vi "Lab Panel V5.27.vi"() -> ()   [LabVIEW 2013] (continued)
                    n2900 = event-data() -> ()  [unwired: 1 in, 6 out]
                    n2901 = Open/Create/Replace File(file path (use dialog)=w5224, operation (0:open)=T17."replace or create") -> (refnum out=w5230:refnum<file>, error out=w5229:errorcluster)  [unwired: 4 in, 1 out]
                    n2902 = Write to Binary File(file (use dialog)=w5230, data=w5225, error in=w5229) -> (refnum out=w5228:refnum<file>, error out=w5227:errorcluster)  [unwired: 3 in, 1 out]
                    n2903 = Close File(refnum=w5228, error in=w5227) -> (error out=w5226:errorcluster)  [unwired: 1 out]
                    n2904 = local write "data file error"(w5226) -> ()
                  }
                  event "MAIL SETTINGS.OUT SERVER ADDRESS", "MAIL SETTINGS.FROM ACCOUNT", "MAIL SETTINGS.USER NAME", "MAIL SETTINGS.PASSWORD", "Auto Mail Send", "TO (string):": Value Change {
                    n2905 = event-data() -> ()  [unwired: 1 in, 6 out]
                    n2906 = local read "MAIL SETTINGS"() -> (w5235:T7)
                    n2907 = local read "Auto Mail Send"() -> (w5233:bool)
                    n2908 = local read "TO (string):"() -> (w5232:string)
                    n2909 = Open/Create/Replace File(file path (use dialog)=w5236, operation (0:open)=T17."replace or create") -> (refnum out=w5241:refnum<file>, error out=w5240:errorcluster)  [unwired: 4 in, 1 out]
                    n2910 = Bundle("MAIL SETTINGS"=w5235, "Auto Mail Send"=w5233, "TO (string):"=w5232) -> (w5234:T43)  [unwired: 1 in]
                    n2911 = Write to Binary File(file (use dialog)=w5241, data=w5234, error in=w5240) -> (refnum out=w5239:refnum<file>, error out=w5238:errorcluster)  [unwired: 3 in, 1 out]
                    n2912 = Close File(refnum=w5239, error in=w5238) -> (error out=w5237:errorcluster)  [unwired: 1 out]
                    n2913 = local write "data file error"(w5237) -> ()
                  }
                }
              }
            }
          }
          frame #19 {
            # "mail control"
            n2914 = local read "MAIL SETTINGS"() -> (w5258:T7)
            n2915 = local read "Auto Mail Send"() -> (w5244:bool)
            n2916 = Unbundle(w5258) -> ("OUT SERVER ADDRESS"=w5257:string, "FROM ACCOUNT"=w5256:string, "TEST MAIL"=w5255:bool)  [unwired: 4 out]
            n2917 = stacked-sequence {
              tunnel: "TO (string):" -> [_ w5297]
              tunnel: w5258 -> [w5263 w5296]
              tunnel: w5257 -> [w5262 w5295]
              tunnel: w5256 -> [w5261 w5294]
              tunnel: w5255 -> [w5260 _]
              tunnel: w5244 -> [_ w5293]
              tunnel: w5254 -> [_ w5292]
              tunnel: w5253 -> [_ w5291]
              tunnel: w5252 -> [_ w5290]
              tunnel: w5251 -> [_ w5289]
              tunnel: w5250 -> [_ w5288]
              tunnel: w5249 -> [_ w5287]
              tunnel: w5248 -> [_ w5286]
              tunnel: w5247 -> [_ w5285]
              tunnel: w5246 -> [_ w5284]
              tunnel: w5245 -> [_ w5283]
              tunnel: "TO (string):" -> [w5259 _]
              frame #0 {
                # "mail test"
                n2918 = case shown="True" w5260 {
                  tunnel: w5263 -> [_ w5267]
                  tunnel: w5259 -> [_ w5266]
                  tunnel: w5262 -> [_ w5265]
                  tunnel: w5261 -> [_ w5264]
                  frame False {
                  }
                  frame True {
                    n2919 = stacked-sequence {
                      seq-local: [_ _ w5277 _] -> [_ _ _ w5278]
                      tunnel: w5267 -> [w5270 _ _ w5282]
                      tunnel: w5266 -> [_ _ w5275 _]
                      tunnel: w5265 -> [_ _ w5273 _]
                      tunnel: w5264 -> [_ _ w5274 _]
                      frame #0 {
                        n2920 = Bundle(cluster=w5270, "TEST MAIL STATUS"="TEST START") -> (w5268:T7)  [unwired: 6 in]
                        n2921 = local write "MAIL SETTINGS"(w5268) -> ()
                      }
                      frame #1 {
                        n2922 = Wait (ms)(milliseconds to wait=500) -> ()  [unwired: 1 out]
                      }
                      frame #2 {
                        n2923 = call "sub vi - send mail v5.vi"("TO:"=w5275, "subject"="MAIL TEST FROM LAB PANEL", "from"=w5274, "out going server"=w5273, "message"="TEST MESSAGE") -> ("error out"=w5277:errorcluster)  [unwired: 10 in]
                      }
                      frame #3 {
                        n2924 = Bundle(cluster=w5282, "TEST MAIL"=FALSE, "TEST MAIL STATUS"="TEST END", "mail error"=w5278) -> (w5280:T7)  [unwired: 4 in]
                        n2925 = local write "MAIL SETTINGS"(w5280) -> ()
                      }
                    }
                  }
                }
              }
              frame #1 {
                # "mail report"
                n2926 = stacked-sequence {
                  seq-local: [_ w5340 _ _] -> [_ _ _ w5530]
                  seq-local: [_ _ w5443 _] -> [_ _ _ w5520]
                  seq-local: [w5307 _ _ _] -> [_ w5357 _ _]
                  seq-local: [w5306 _ _ _] -> [_ w5356 _ _]
                  seq-local: [w5304 _ _ _] -> [_ w5354 _ _]
                  seq-local: [w5305 _ _ _] -> [_ w5355 _ _]
                  seq-local: [w5303 _ _ _] -> [_ w5353 _ _]
                  seq-local: [w5302 _ _ _] -> [_ w5348 _ _]
                  seq-local: [w5301 _ _ _] -> [_ w5349 _ _]
                  seq-local: [w5300 _ _ _] -> [_ w5350 _ _]
                  seq-local: [w5299 _ _ _] -> [_ w5351 _ _]
                  seq-local: [w5298 _ _ _] -> [_ w5352 _ _]
                  tunnel: w5297 -> [_ _ _ w5531]
                  tunnel: w5296 -> [_ _ _ w5514]
                  tunnel: w5295 -> [_ _ _ w5528]
                  tunnel: w5294 -> [_ _ _ w5527]
                  tunnel: w5293 -> [w5338 _ _ w5522]
                  tunnel: w5292 -> [_ _ w5473 _]
                  tunnel: w5291 -> [_ _ w5470 _]
                  tunnel: w5290 -> [_ _ w5469 _]
                  tunnel: w5289 -> [_ _ w5468 _]
                  tunnel: w5288 -> [_ _ w5467 _]
                  tunnel: w5287 -> [_ _ w5466 _]
                  tunnel: w5286 -> [_ _ w5465 _]
                  tunnel: w5285 -> [_ _ w5464 _]
                  tunnel: w5284 -> [_ _ w5463 _]
                  tunnel: w5283 -> [_ _ w5462 _]
                  frame #0 {
                    n2927 = case shown="False" w5338 {
                      frame False {
                        n2928 = local write "mail control"("") -> ()
                      }
                      frame True {
                      }
                    }
                    n2929 = local read "SET LAB01-1"() -> (w5337:T5)
                    n2930 = local read "SET LAB01-2"() -> (w5336:T5)
                    n2931 = local read "SET LAB02-1"() -> (w5335:T5)
                    n2932 = local read "SET LAB02-2"() -> (w5334:T5)
                    n2933 = local read "SET LAB03-1"() -> (w5333:T5)
                    n2934 = local read "SET LAB04-1"() -> (w5331:T5)
                    n2935 = local read "SET LAB05-1"() -> (w5329:T5)
                    n2936 = local read "SET LAB03-2"() -> (w5332:T5)
                    n2937 = local read "SET LAB04-2"() -> (w5330:T5)
                    n2938 = local read "SET LAB05-2"() -> (w5328:T5)
                    n2939 = Unbundle(w5333) -> ("DESCRIPTION"=w5313:string)  [unwired: 4 out]
                    n2940 = Unbundle(w5332) -> ("DESCRIPTION"=w5312:string)  [unwired: 4 out]
                    n2941 = Unbundle(w5331) -> ("DESCRIPTION"=w5311:string)  [unwired: 4 out]
                    n2942 = Unbundle(w5328) -> ("DESCRIPTION"=w5308:string)  [unwired: 4 out]
                    n2943 = Unbundle(w5334) -> ("DESCRIPTION"=w5314:string)  [unwired: 4 out]
                    n2944 = Unbundle(w5330) -> ("DESCRIPTION"=w5310:string)  [unwired: 4 out]
                    n2945 = Unbundle(w5337) -> ("DESCRIPTION"=w5326:string)  [unwired: 4 out]
                    n2946 = Unbundle(w5335) -> ("DESCRIPTION"=w5315:string)  [unwired: 4 out]
                    n2947 = Unbundle(w5329) -> ("DESCRIPTION"=w5309:string)  [unwired: 4 out]
                    n2948 = Unbundle(w5336) -> ("DESCRIPTION"=w5316:string)  [unwired: 4 out]
                    n2949 = Concatenate Strings("[LAB05-2/", w5308) -> (w5298:string)
                    n2950 = Concatenate Strings("[LAB05-1/", w5309) -> (w5299:string)
                    n2951 = Concatenate Strings("[LAB04-2/", w5310) -> (w5300:string)
                    n2952 = Concatenate Strings("[LAB03-2/", w5312) -> (w5302:string)
                    n2953 = Concatenate Strings("[LAB04-1/", w5311) -> (w5301:string)
                    n2954 = Concatenate Strings("[LAB03-1/", w5313) -> (w5303:string)
                    n2955 = Concatenate Strings("[LAB01-2/", w5316) -> (w5306:string)
                    n2956 = Concatenate Strings("[LAB02-2/", w5314) -> (w5304:string)
                    n2957 = Concatenate Strings("[LAB01-1/", w5326) -> (w5307:string)
                    n2958 = Concatenate Strings("[LAB02-1/", w5315) -> (w5305:string)
                  }
                  frame #1 {
                    w5361 = "/"
                    w5362 = 2.0
                    n2959 = local read "DISP LAB01-2"() -> (w5441:T4)
                    n2960 = local read "DISP LAB01-1"() -> (w5442:T4)
                    n2961 = local read "DISP LAB02-1"() -> (w5440:T4)
                    n2962 = local read "DISP LAB03-2"() -> (w5437:T4)
                    n2963 = local read "DISP LAB02-2"() -> (w5439:T4)
                    n2964 = local read "DISP LAB03-1"() -> (w5438:T4)
                    n2965 = local read "DISP LAB04-2"() -> (w5435:T4)
                    n2966 = local read "DISP LAB04-1"() -> (w5436:T4)
                    n2967 = local read "DISP LAB05-1"() -> (w5434:T4)
                    n2968 = local read "DISP LAB05-2"() -> (w5433:T4)
                    n2969 = Unbundle(w5441) -> ("CYCLE"=w5425:dbl, "MINS"=w5424:dbl, "STATUS"=w5421:string)
                    n2970 = Unbundle(w5442) -> ("CYCLE"=w5430:dbl, "MINS"=w5429:dbl, "STATUS"=w5426:string)
                    n2971 = Unbundle(w5440) -> ("CYCLE"=w5418:dbl, "MINS"=w5417:dbl, "STATUS"=w5416:string)
                    n2972 = Unbundle(w5437) -> ("CYCLE"=w5405:dbl, "MINS"=w5404:dbl, "STATUS"=w5401:string)
                    n2973 = Unbundle(w5438) -> ("CYCLE"=w5410:dbl, "MINS"=w5409:dbl, "STATUS"=w5406:string)
                    n2974 = Unbundle(w5439) -> ("CYCLE"=w5415:dbl, "MINS"=w5414:dbl, "STATUS"=w5411:string)
                    n2975 = Unbundle(w5436) -> ("CYCLE"=w5400:dbl, "MINS"=w5399:dbl, "STATUS"=w5396:string)
                    n2976 = Unbundle(w5435) -> ("CYCLE"=w5395:dbl, "MINS"=w5394:dbl, "STATUS"=w5391:string)
                    n2977 = Unbundle(w5434) -> ("CYCLE"=w5390:dbl, "MINS"=w5389:dbl, "STATUS"=w5386:string)
                    n2978 = Unbundle(w5433) -> ("CYCLE"=w5432:dbl, "MINS"=w5431:dbl, "STATUS"=w5383:string)
                    n2979 = Number To Decimal String(number=w5418) -> (decimal integer string=w5420:string)  [unwired: 1 in]
                    n2980 = Number To Decimal String(number=w5415) -> (decimal integer string=w5413:string)  [unwired: 1 in]
                    n2981 = Number To Decimal String(number=w5410) -> (decimal integer string=w5408:string)  [unwired: 1 in]
                    n2982 = Number To Decimal String(number=w5425) -> (decimal integer string=w5423:string)  [unwired: 1 in]
                    n2983 = Number To Decimal String(number=w5405) -> (decimal integer string=w5403:string)  [unwired: 1 in]
                    n2984 = Number To Decimal String(number=w5430) -> (decimal integer string=w5428:string)  [unwired: 1 in]
                    n2985 = Number To Decimal String(number=w5432) -> (decimal integer string=w5385:string)  [unwired: 1 in]
                    n2986 = Number To Decimal String(number=w5400) -> (decimal integer string=w5398:string)  [unwired: 1 in]
                    n2987 = Number To Decimal String(number=w5395) -> (decimal integer string=w5393:string)  [unwired: 1 in]
                    n2988 = Number To Decimal String(number=w5390) -> (decimal integer string=w5388:string)  [unwired: 1 in]
                    n2989 = Number To Fractional String(number=w5417, precision (6)=w5362) -> (F-format string=w5419:string)  [unwired: 2 in]
                    n2990 = Number To Fractional String(number=w5404, precision (6)=w5362) -> (F-format string=w5402:string)  [unwired: 2 in]
                    n2991 = Number To Fractional String(number=w5414, precision (6)=w5362) -> (F-format string=w5412:string)  [unwired: 2 in]
                    n2992 = Number To Fractional String(number=w5409, precision (6)=w5362) -> (F-format string=w5407:string)  [unwired: 2 in]
                    n2993 = Number To Fractional String(number=w5394, precision (6)=w5362) -> (F-format string=w5392:string)  [unwired: 2 in]
                    n2994 = Number To Fractional String(number=w5399, precision (6)=w5362) -> (F-format string=w5397:string)  [unwired: 2 in]
                    n2995 = Number To Fractional String(number=w5424, precision (6)=w5362) -> (F-format string=w5422:string)  [unwired: 2 in]
                    n2996 = Number To Fractional String(number=w5389, precision (6)=w5362) -> (F-format string=w5387:string)  [unwired: 2 in]
                    n2997 = Number To Fractional String(number=w5429, precision (6)=w5362) -> (F-format string=w5427:string)  [unwired: 2 in]
                    n2998 = Number To Fractional String(number=w5431, precision (6)=w5362) -> (F-format string=w5384:string)  [unwired: 2 in]
                    n2999 = Concatenate Strings(w5361, w5403, w5361, w5402, w5361, w5401) -> (w5377:string)
                    n3000 = Concatenate Strings(w5361, w5398, w5361, w5397, w5361, w5396) -> (w5376:string)
                    n3001 = Concatenate Strings(w5361, w5393, w5361, w5392, w5361, w5391) -> (w5375:string)
                    n3002 = Concatenate Strings(w5361, w5388, w5361, w5387, w5361, w5386) -> (w5374:string)
                    n3003 = Concatenate Strings(w5361, w5385, w5361, w5384, w5361, w5383) -> (w5373:string)
                    n3004 = Concatenate Strings(w5361, w5428, w5361, w5427, w5361, w5426) -> (w5382:string)
                    n3005 = Concatenate Strings(w5361, w5408, w5361, w5407, w5361, w5406) -> (w5378:string)
                    n3006 = Concatenate Strings(w5361, w5423, w5361, w5422, w5361, w5421) -> (w5381:string)
                    n3007 = Concatenate Strings(w5361, w5420, w5361, w5419, w5361, w5416) -> (w5380:string)
                    n3008 = Concatenate Strings(w5361, w5413, w5361, w5412, w5361, w5411) -> (w5379:string)
                    n3009 = Concatenate Strings("]", "\r") -> (w5358:string)
                    n3010 = Concatenate Strings(w5353, w5378, w5358) -> (w5368:string)
                    n3011 = Concatenate Strings(w5355, w5380, w5358) -> (w5370:string)
                    n3012 = Concatenate Strings(w5354, w5379, w5358) -> (w5369:string)
                    n3013 = Concatenate Strings(w5350, w5375, w5358) -> (w5365:string)
                    n3014 = Concatenate Strings(w5351, w5374, w5358) -> (w5366:string)
                    n3015 = Concatenate Strings(w5349, w5376, w5358) -> (w5364:string)
                    n3016 = Concatenate Strings(w5348, w5377, w5358) -> (w5363:string)
                    n3017 = Concatenate Strings(w5352, w5373, w5358) -> (w5367:string)
                    n3018 = Concatenate Strings(w5356, w5381, w5358) -> (w5371:string)
                    n3019 = Concatenate Strings(w5357, w5382, w5358) -> (w5372:string)
                    n3020 = Concatenate Strings(w5372, w5371, w5370, w5369, w5368, w5363, w5364, w5365, w5366, w5367) -> (w5341:string)
                    n3021 = Concatenate Strings("[PANEL/", "DESC/", "CYCLES/", "MINS/", "STATUS]", "\r", w5341) -> (w5340:string)
                    "MAIL REPORT" <- w5340
                    n3022 = global write "Global display 3.vi" "log all"(w5340) -> ()
                  }
                  frame #2 {
                    w5471 = "END"
                    n3023 = local read "mail control"() -> (w5472:string)
                    n3024 = case shown="False" w5467 {
                      tunnel: w5472 -> [w5496 _]
                      tunnel: w5471 -> [w5495 _]
                      tunnel: [w5494 FALSE] -> w5457
                      frame False {
                        n3025 = Equal?(x=w5496, y=w5495) -> (x = y?=w5494:bool)
                      }
                      frame True {
                      }
                    }
                    n3026 = case shown="False" w5473 {
                      tunnel: w5472 -> [w5512 _]
                      tunnel: w5471 -> [w5511 _]
                      tunnel: [w5510 FALSE] -> w5461
                      frame False {
                        n3027 = Equal?(x=w5512, y=w5511) -> (x = y?=w5510:bool)
                      }
                      frame True {
                      }
                    }
                    n3028 = case shown="False" w5470 {
                      tunnel: w5472 -> [w5508 _]
                      tunnel: w5471 -> [w5507 _]
                      tunnel: [w5506 FALSE] -> w5460
                      frame False {
                        n3029 = Equal?(x=w5508, y=w5507) -> (x = y?=w5506:bool)
                      }
                      frame True {
                      }
                    }
                    n3030 = case shown="False" w5468 {
                      tunnel: w5472 -> [w5500 _]
                      tunnel: w5471 -> [w5499 _]
                      tunnel: [w5498 FALSE] -> w5458
                      frame False {
                        n3031 = Equal?(x=w5500, y=w5499) -> (x = y?=w5498:bool)
                      }
                      frame True {
                      }
                    }
                    n3032 = case shown="False" w5469 {
                      tunnel: w5472 -> [w5504 _]
                      tunnel: w5471 -> [w5503 _]
                      tunnel: [w5502 FALSE] -> w5459
                      frame False {
                        n3033 = Equal?(x=w5504, y=w5503) -> (x = y?=w5502:bool)
                      }
                      frame True {
                      }
                    }
                    n3034 = Or(x=w5459, y=w5458) -> (x .or. y?=w5450:bool)
                    n3035 = Or(x=w5461, y=w5460) -> (x .or. y?=w5451:bool)
                    n3036 = Or(x=w5451, y=w5450) -> (x .or. y?=w5446:bool)
                    n3037 = case shown="False" w5463 {
                      tunnel: w5472 -> [w5480 _]
                      tunnel: w5471 -> [w5479 _]
                      tunnel: [w5478 FALSE] -> w5452
                      frame False {
                        n3038 = Equal?(x=w5480, y=w5479) -> (x = y?=w5478:bool)
                      }
                      frame True {
                      }
                    }
                    n3039 = case shown="False" w5462 {
                      tunnel: w5472 -> [w5476 _]
                      tunnel: w5471 -> [w5475 _]
                      tunnel: [w5474 FALSE] -> w5456
                      frame False {
                        n3040 = Equal?(x=w5476, y=w5475) -> (x = y?=w5474:bool)
                      }
                      frame True {
                      }
                    }
                    n3041 = case shown="False" w5464 {
                      tunnel: w5472 -> [w5484 _]
                      tunnel: w5471 -> [w5483 _]
                      tunnel: [w5482 FALSE] -> w5453
                      frame False {
                        n3042 = Equal?(x=w5484, y=w5483) -> (x = y?=w5482:bool)
                      }
                      frame True {
                      }
                    }
                    n3043 = case shown="False" w5466 {
                      tunnel: w5472 -> [w5492 _]
                      tunnel: w5471 -> [w5491 _]
                      tunnel: [w5490 FALSE] -> w5455
                      frame False {
                        n3044 = Equal?(x=w5492, y=w5491) -> (x = y?=w5490:bool)
                      }
                      frame True {
                      }
                    }
                    n3045 = case shown="False" w5465 {
                      tunnel: w5472 -> [w5488 _]
                      tunnel: w5471 -> [w5487 _]
                      tunnel: [w5486 FALSE] -> w5454
                      frame False {
                        n3046 = Equal?(x=w5488, y=w5487) -> (x = y?=w5486:bool)
                      }
                      frame True {
                      }
                    }
                    n3047 = Or(x=w5455, y=w5454) -> (x .or. y?=w5449:bool)
                    n3048 = Or(x=w5453, y=w5452) -> (x .or. y?=w5448:bool)
                    n3049 = Or(x=w5456, y=w5457) -> (x .or. y?=w5444:bool)
                    n3050 = Or(x=w5449, y=w5448) -> (x .or. y?=w5447:bool)
                    n3051 = Or(x=w5446, y=w5447) -> (x .or. y?=w5445:bool)
                    n3052 = Or(x=w5445, y=w5444) -> (x .or. y?=w5443:bool)
                  }
                  frame #3 {
                    n3053 = local read "on loops"() -> (w5526:dbl)
                    n3054 = local read "jig cycle"() -> (w5523:dbl)
                    n3055 = local read "Send Mail Now"() -> (w5517:bool)
                    n3056 = Add(x=w5526, y=5.0) -> (x+y=w5524:dbl)
                    n3057 = Equal?(x=w5523, y=w5524) -> (x = y?=w5518:bool)
                    n3058 = And(x=w5518, y=w5517) -> (x .and. y?=w5516:bool)
                    n3059 = And(x=w5522, y=w5518) -> (x .and. y?=w5521:bool)
                    n3060 = And(x=w5521, y=w5520) -> (x .and. y?=w5519:bool)
                    n3061 = Or(x=w5519, y=w5516) -> (x .or. y?=w5515:bool)
                    n3062 = case shown="True" w5515 {
                      tunnel: w5531 -> [_ w5537]
                      tunnel: w5530 -> [_ w5536]
                      tunnel: "Lab Panel Test Status" -> [_ w5535]
                      tunnel: w5528 -> [_ w5534]
                      tunnel: w5527 -> [_ w5533]
                      tunnel: w5514 -> [_ w5532]
                      frame False {
                      }
                      frame True {
                        n3063 = stacked-sequence {
                          tunnel: w5537 -> [w5546 _]
                          tunnel: w5536 -> [w5545 _]
                          tunnel: w5535 -> [w5544 _]
                          tunnel: w5534 -> [w5543 _]
                          tunnel: w5533 -> [w5542 _]
                          tunnel: w5532 -> [w5541 _]
                          frame #0 {
                            n3064 = call "sub vi - send mail v5.vi"("TO:"=w5546, "subject"=w5544, "Info"="Test station status report", "from"=w5542, "out going server"=w5543, "message"=w5545) -> ("error out"=w5540:errorcluster)  [unwired: 9 in]
                            n3065 = Bundle(cluster=w5541, "mail error"=w5540) -> (w5539:T7)  [unwired: 6 in]
                            n3066 = local write "MAIL SETTINGS"(w5539) -> ()
                          }
                          frame #1 {
                            n3067 = local write "mail control"("") -> ()
                            n3068 = local write "Send Mail Now"(FALSE) -> ()
                          }
                        }
                      }
                    }
                  }
                }
              }
            }
          }
          frame #20 {
            # "save jig cycle values once all run switches are off"
            n3069 = stacked-sequence {
              tunnel: w5558 -> [_ w5587]
              tunnel: w5557 -> [_ w5586]
              tunnel: w5556 -> [_ w5585]
              tunnel: w5555 -> [_ w5584]
              tunnel: w5554 -> [_ w5583]
              tunnel: w5553 -> [_ w5582]
              tunnel: w5552 -> [_ w5581]
              tunnel: w5551 -> [_ w5580]
              tunnel: w5550 -> [_ w5579]
              tunnel: w5549 -> [_ w5578]
              frame #0 {
              }
              frame #1 {
                n3070 = Not(x=w5578) -> (.not. x?=w5561:bool)
                n3071 = Not(x=w5586) -> (.not. x?=w5576:bool)
                n3072 = Not(x=w5583) -> (.not. x?=w5571:bool)
                n3073 = Not(x=w5581) -> (.not. x?=w5567:bool)
                n3074 = Not(x=w5579) -> (.not. x?=w5563:bool)
                n3075 = Not(x=w5587) -> (.not. x?=w5577:bool)
                n3076 = Not(x=w5585) -> (.not. x?=w5575:bool)
                n3077 = Not(x=w5582) -> (.not. x?=w5569:bool)
                n3078 = Not(x=w5584) -> (.not. x?=w5573:bool)
                n3079 = Not(x=w5580) -> (.not. x?=w5565:bool)
                n3080 = local read "Save JC"() -> (w5589:bool)
                n3081 = And(x=w5577, y=w5576) -> (x .and. y?=w5574:bool)
                n3082 = And(x=w5574, y=w5575) -> (x .and. y?=w5572:bool)
                n3083 = And(x=w5572, y=w5573) -> (x .and. y?=w5570:bool)
                n3084 = And(x=w5570, y=w5571) -> (x .and. y?=w5568:bool)
                n3085 = And(x=w5568, y=w5569) -> (x .and. y?=w5566:bool)
                n3086 = And(x=w5566, y=w5567) -> (x .and. y?=w5564:bool)
                n3087 = And(x=w5564, y=w5565) -> (x .and. y?=w5562:bool)
                n3088 = And(x=w5562, y=w5563) -> (x .and. y?=w5560:bool)
                n3089 = And(x=w5560, y=w5561) -> (x .and. y?=w5559:bool)
                n3090 = And(x=w5559, y=w5589) -> (x .and. y?=w5588:bool)
                n3091 = case shown="True" w5588 {
                  tunnel: w5559 -> [w5590 _]
                  frame False {
                    n3092 = case shown="False" w5590 {
                      frame False {
                        n3093 = local write "Save JC"(TRUE) -> ()
                      }
                      frame True {
                      }
                    }
                  }
                  frame True {
                    n3094 = stacked-sequence {
                      frame #0 {
                        n3095 = String To Path(string="c:\\crabtree\\Jig Cycles\\") -> (path=w5602:path)
                        n3096 = Build Path(base path=w5602, name or relative path="jigcycles.bin") -> (appended path=w5600:path)
                        n3097 = Create Folder(path (use dialog)=w5602) -> (error out=w5604:errorcluster)  [unwired: 2 in, 2 out]
                        n3098 = local read "JIG RELAY CYCLES"() -> (w5594:T8)
                        n3099 = call <vilib>:"Clear Errors.vi"("error in (no error)"=w5604) -> ()  [unwired: 6 in, 1 out]
                        n3100 = local write "Save JC"(FALSE) -> ()
                        n3101 = Open/Create/Replace File(file path (use dialog)=w5600, operation (0:open)=T17."replace or create") -> (refnum out=w5598:refnum<file>, error out=w5599:errorcluster)  [unwired: 4 in, 1 out]
                        n3102 = Write to Binary File(file (use dialog)=w5598, data=w5594, error in=w5599) -> (refnum out=w5597:refnum<file>, error out=w5596:errorcluster)  [unwired: 3 in, 1 out]
                        n3103 = Close File(refnum=w5597, error in=w5596) -> (error out=w5595:errorcluster)  [unwired: 1 out]
                        n3104 = local write "data file error"(w5595) -> ()
                      }
                      frame #1 {
                        n3105 = local read "JIG RELAY CYCLES"() -> (w5627:T8)
                        n3106 = Unbundle By Name(w5627) -> ("LAB01-1"=w5622:dbl, "LAB01-2"=w5621:dbl, "LAB02-1"=w5619:dbl, "LAB02-2"=w5618:dbl, "LAB03-1"=w5616:dbl, "LAB03-2"=w5613:dbl, "LAB04-1"=w5612:dbl, "LAB04-2"=w5610:dbl, "LAB05-1"=w5608:dbl, "LAB05-2"=w5606:dbl)
                        n3107 = stacked-sequence {
                          tunnel: w5622 -> [w5630 _ _ _ _ _ _ _ _ _]
                          tunnel: 1000000 -> [w5633 w5643 w5653 w5663 w5673 w5683 w5693 w5703 w5713 w5723]
                          tunnel: [w5631 _ _ _ _ _ _ _ _ _] -> w5625
                          tunnel: "TEST STATION HAS REACHED 1 MILLION CYCLES, REPLACE  CONTROL RELAYS" -> [w5629 w5641 w5651 w5661 w5671 w5681 w5691 w5701 w5711 w5721]
                          tunnel: [_ w5640 _ _ _ _ _ _ _ _] -> w5623
                          tunnel: w5621 -> [_ w5639 _ _ _ _ _ _ _ _]
                          tunnel: [_ _ w5650 _ _ _ _ _ _ _] -> w5620
                          tunnel: w5619 -> [_ _ w5649 _ _ _ _ _ _ _]
                          tunnel: w5618 -> [_ _ _ w5660 _ _ _ _ _ _]
                          tunnel: [_ _ _ w5659 _ _ _ _ _ _] -> w5617
                          tunnel: w5616 -> [_ _ _ _ w5670 _ _ _ _ _]
                          tunnel: [_ _ _ _ w5669 _ _ _ _ _] -> w5615
                          tunnel: [_ _ _ _ _ w5680 _ _ _ _] -> w5614
                          tunnel: w5613 -> [_ _ _ _ _ w5679 _ _ _ _]
                          tunnel: w5612 -> [_ _ _ _ _ _ w5690 _ _ _]
                          tunnel: [_ _ _ _ _ _ w5689 _ _ _] -> w5611
                          tunnel: w5610 -> [_ _ _ _ _ _ _ w5700 _ _]
                          tunnel: [_ _ _ _ _ _ _ w5699 _ _] -> w5609
                          tunnel: w5608 -> [_ _ _ _ _ _ _ _ w5710 _]
                          tunnel: [_ _ _ _ _ _ _ _ w5709 _] -> w5607
                          tunnel: w5606 -> [_ _ _ _ _ _ _ _ _ w5720]
                          tunnel: [_ _ _ _ _ _ _ _ _ w5719] -> w5605
                          frame #0 {
                            n3108 = Greater?(x=w5630, y=w5633) -> (0:w5632:bool)
                            n3109 = case shown="True" w5632 {
                              tunnel: [w5634 0] -> w5631
                              tunnel: w5630 -> [w5634 _]
                              tunnel: w5629 -> [_ w5635]
                              frame False {
                              }
                              frame True {
                                n3110 = Concatenate Strings("LA01-1 ", w5635) -> (w5638:string)
                                n3111 = One Button Dialog(message=w5638) -> ()  [unwired: 1 in, 1 out]
                              }
                            }
                          }
                          frame #1 {
                            n3112 = Greater?(x=w5639, y=w5643) -> (0:w5642:bool)
                            n3113 = case shown="True" w5642 {
                              tunnel: [w5644 0] -> w5640
                              tunnel: w5639 -> [w5644 _]
                              tunnel: w5641 -> [_ w5645]
                              frame False {
                              }
                              frame True {
                                n3114 = Concatenate Strings("LA01-2 ", w5645) -> (w5648:string)
                                n3115 = One Button Dialog(message=w5648) -> ()  [unwired: 1 in, 1 out]
                              }
                            }
                          }
                          frame #2 {
                            n3116 = Greater?(x=w5649, y=w5653) -> (0:w5652:bool)
                            n3117 = case shown="True" w5652 {
                              tunnel: [w5654 0] -> w5650
                              tunnel: w5649 -> [w5654 _]
                              tunnel: w5651 -> [_ w5655]
                              frame False {
                              }
                              frame True {
                                n3118 = Concatenate Strings("LA02-1 ", w5655) -> (w5658:string)
                                n3119 = One Button Dialog(message=w5658) -> ()  [unwired: 1 in, 1 out]
                              }
                            }
                          }
                          frame #3 {
                            n3120 = Greater?(x=w5660, y=w5663) -> (0:w5662:bool)
                            n3121 = case shown="True" w5662 {
                              tunnel: [w5664 0] -> w5659
                              tunnel: w5660 -> [w5664 _]
                              tunnel: w5661 -> [_ w5665]
                              frame False {
                              }
                              frame True {
                                n3122 = Concatenate Strings("LA02-2 ", w5665) -> (w5668:string)
                                n3123 = One Button Dialog(message=w5668) -> ()  [unwired: 1 in, 1 out]
                              }
                            }
                          }
                          frame #4 {
                            n3124 = Greater?(x=w5670, y=w5673) -> (0:w5672:bool)
                            n3125 = case shown="True" w5672 {
                              tunnel: [w5674 0] -> w5669
                              tunnel: w5670 -> [w5674 _]
                              tunnel: w5671 -> [_ w5675]
                              frame False {
                              }
                              frame True {
                                n3126 = Concatenate Strings("LA03-1 ", w5675) -> (w5678:string)
                                n3127 = One Button Dialog(message=w5678) -> ()  [unwired: 1 in, 1 out]
                              }
                            }
                          }
                          frame #5 {
                            n3128 = Greater?(x=w5679, y=w5683) -> (0:w5682:bool)
                            n3129 = case shown="True" w5682 {
                              tunnel: [w5684 0] -> w5680
                              tunnel: w5679 -> [w5684 _]
                              tunnel: w5681 -> [_ w5685]
                              frame False {
                              }
                              frame True {
                                n3130 = Concatenate Strings("LA03-2 ", w5685) -> (w5688:string)
                                n3131 = One Button Dialog(message=w5688) -> ()  [unwired: 1 in, 1 out]
                              }
                            }
                          }
                          frame #6 {
                            n3132 = Greater?(x=w5690, y=w5693) -> (0:w5692:bool)
                            n3133 = case shown="True" w5692 {
                              tunnel: [w5694 0] -> w5689
                              tunnel: w5690 -> [w5694 _]
                              tunnel: w5691 -> [_ w5695]
                              frame False {
                              }
                              frame True {
                                n3134 = Concatenate Strings("LA04-1 ", w5695) -> (w5698:string)
                                n3135 = One Button Dialog(message=w5698) -> ()  [unwired: 1 in, 1 out]
                              }
                            }
                          }
                          frame #7 {
                            n3136 = Greater?(x=w5700, y=w5703) -> (0:w5702:bool)
                            n3137 = case shown="True" w5702 {
                              tunnel: [w5704 0] -> w5699
                              tunnel: w5700 -> [w5704 _]
                              tunnel: w5701 -> [_ w5705]
                              frame False {
                              }
                              frame True {
                                n3138 = Concatenate Strings("LA04-2 ", w5705) -> (w5708:string)
                                n3139 = One Button Dialog(message=w5708) -> ()  [unwired: 1 in, 1 out]
                              }
                            }
                          }
                          frame #8 {
                            n3140 = Greater?(x=w5710, y=w5713) -> (0:w5712:bool)
                            n3141 = case shown="True" w5712 {
                              tunnel: [w5714 0] -> w5709
                              tunnel: w5710 -> [w5714 _]
                              tunnel: w5711 -> [_ w5715]
                              frame False {
                              }
                              frame True {
                                n3142 = Concatenate Strings("LA05-1 ", w5715) -> (w5718:string)
                                n3143 = One Button Dialog(message=w5718) -> ()  [unwired: 1 in, 1 out]
                              }
                            }
                          }
                          frame #9 {
                            n3144 = Greater?(x=w5720, y=w5723) -> (0:w5722:bool)
                            n3145 = case shown="True" w5722 {
                              tunnel: [w5724 0] -> w5719
                              tunnel: w5720 -> [w5724 _]
                              tunnel: w5721 -> [_ w5725]
                              frame False {
                              }
                              frame True {
                                n3146 = Concatenate Strings("LA05-2 ", w5725) -> (w5728:string)
                                n3147 = One Button Dialog(message=w5728) -> ()  [unwired: 1 in, 1 out]
                              }
                            }
                          }
                        }
                        n3148 = Bundle By Name(cluster=w5627, "LAB01-1"=w5625, "LAB01-2"=w5623, "LAB02-1"=w5620, "LAB02-2"=w5617, "LAB03-1"=w5615, "LAB03-2"=w5614, "LAB04-1"=w5611, "LAB04-2"=w5609, "LAB05-1"=w5607, "LAB05-2"=w5605) -> (w5626:T8)
                        n3149 = local write "JIG RELAY CYCLES"(w5626) -> ()
                      }
                    }
                  }
                }
              }
            }
          }
          frame #21 {
            # "get temperature values"
            n3150 = local read "Simulate"() -> (w5741:bool)
            n3151 = local read "Temp Test Cal"() -> (w5738:dbl)
            n3152 = stacked-sequence {
              seq-local: [w5743 _] -> [_ w5788]
              tunnel: w5741 -> [_ w5801]
              tunnel: T14 {"1  (A) cal"=1.0, "1 (V) cal"=1.0, "1 (PF) cal"=1.0, "1 (TL) cal"=1.0, "1 (TN) cal"=1.0, "2 (A) cal"=1.0, "2 (V) cal"=1.0, "2 (PF) cal"=1.0, "2 (TL) cal"=1.0, "2 (TN) cal"=1.0} ("CAL LAB01") -> [_ w5800]
              tunnel: w5739 -> [_ w5799]
              tunnel: w5738 -> [_ w5798]
              tunnel: w5737 -> [_ w5797]
              tunnel: w5736 -> [_ w5796]
              tunnel: w5735 -> [_ w5795]
              tunnel: w5734 -> [_ w5794]
              tunnel: w5733 -> [_ w5793]
              tunnel: w5732 -> [_ w5792]
              tunnel: w5731 -> [_ w5791]
              tunnel: w5730 -> [_ w5790]
              tunnel: w5729 -> [_ w5789]
              frame #0 {
                # "only get temperature from initial valid temperature circuits"
                n3153 = local read "Select COM port"() -> (w5751:refnum<visa-resource-name>)
                "COM port" <- w5751
                n3154 = global write "Global 1.vi" "COM port"(w5751) -> ()
                n3155 = local read "Temp read loop"() -> (w5748:dbl)
                n3156 = global write "Global 1.vi" "tmp dly lps"("Temp Delay Lps") -> ()
                n3157 = global write "Global 1.vi" "dly value"("Temp Value") -> ()
                n3158 = local read "jig cycle"() -> (w5752:dbl)
                n3159 = local read "on loops"() -> (w5754:dbl)
                n3160 = Equal?(x=w5748, y=1) -> (x = y?=w5745:bool)
                n3161 = Add(x=w5754, y=6) -> (x+y=w5755:dbl)
                n3162 = Equal?(x=w5752, y=w5755) -> (x = y?=w5746:bool)
                n3163 = And(x=w5746, y=w5745) -> (x .and. y?=w5744:bool)
                n3164 = Or(x=w5744, y="Read Temp") -> (x .or. y?=w5743:bool)
                n3165 = case shown="True" w5743 {
                  frame False {
                  }
                  frame True {
                    n3166 = local read "Simulate"() -> (w5757:bool)
                    n3167 = local write "TEMP"(TRUE) -> ()
                    n3168 = local write "Read Temp"(FALSE) -> ()
                    n3169 = stacked-sequence {
                      tunnel: 1.0 -> [_ _ _ _ w5787]
                      tunnel: w5757 -> [_ _ _ _ w5786]
                      frame #0 {
                        # "only switch relay on to reset temp circuits if busy testing"
                        n3170 = disable-structure shown="Disabled" {
                          frame Disabled {
                            n3171 = local read "Any Test Running"() -> ()  [unwired: 1 out]
                          }
                          frame Enabled {
                          }
                        }
                        n3172 = local read "USB OUT 0"() -> (w5761:bool[])
                        n3173 = local read "USB OUT 2"() -> (w5763:bool[])
                        n3174 = local read "USB OUT 1"() -> (w5762:bool[])
                        n3175 = Insert Into Array(array=w5763, index=7, new element=TRUE) -> (w5764:bool[])
                        n3176 = call "sub vi - Drive Relays All v6.vi"("Array #2"=w5764, "Array #1"=w5762, "Array #0"=w5761) -> ()  [unwired: 8 in, 1 out]
                      }
                      frame #1 {
                        # "time delay"
                        n3177 = Wait (ms)(milliseconds to wait=500) -> ()  [unwired: 1 out]
                      }
                      frame #2 {
                        # "switch relay off"
                        n3178 = local read "USB OUT 0"() -> (w5767:bool[])
                        n3179 = local read "USB OUT 2"() -> (w5769:bool[])
                        n3180 = local read "USB OUT 1"() -> (w5768:bool[])
                        n3181 = Insert Into Array(array=w5769, index=7, new element=FALSE) -> (w5770:bool[])
                        n3182 = call "sub vi - Drive Relays All v6.vi"("Array #2"=w5770, "Array #1"=w5768, "Array #0"=w5767) -> ()  [unwired: 8 in, 1 out]
                      }
                      frame #3 {
                        # "time delay"
                        n3183 = Wait (ms)(milliseconds to wait=300) -> ()  [unwired: 1 out]
                      }
                      frame #4 {
                        # "read all valid temp circuits"
                        n3184 = local read "LAB01-TP"() -> (w5779:bool)
                        n3185 = local read "LAB03-TP"() -> (w5777:bool)
                        n3186 = local read "LAB02-TP"() -> (w5778:bool)
                        n3187 = local read "LAB04-TP"() -> (w5776:bool)
                        n3188 = local read "LAB05-TP"() -> (w5780:bool)
                        n3189 = call "sub vi - GET ALL TEMP v7.vi"("LA01-EN"=w5779, "simulate"=w5786, "LA02-EN"=w5778, "LA03-EN"=w5777, "LA04-EN"=w5776, "LA05-EN"=w5780, "Gen Cal Value"=w5787) -> ("LOOP TIME"=→"Read Time":dbl, "LA01 TEMP"=w5785:T25, "LA02 TEMP"=w5784:T25, "LA03 TEMP"=w5783:T25, "LA04 TEMP"=w5782:T25, "error"=→"Error Temp":bool, "LA05 TEMP"=w5781:T25)  [unwired: 1 in, 1 out]
                        n3190 = local write "LAB01 TEMP"(w5785) -> ()
                        n3191 = local write "LAB02 TEMP"(w5784) -> ()
                        n3192 = local write "LAB03 TEMP"(w5783) -> ()
                        n3193 = local write "LAB04 TEMP"(w5782) -> ()
                        n3194 = local write "LAB05 TEMP"(w5781) -> ()
                      }
                    }
                  }
                }
              }
              frame #1 {
                n3195 = case shown="True" w5788 {
                  tunnel: w5801 -> [_ w5814]
                  tunnel: w5800 -> [_ w5813]
                  tunnel: w5799 -> [_ w5812]
                  tunnel: w5798 -> [_ w5811]
                  tunnel: w5797 -> [_ w5810]
                  tunnel: w5796 -> [_ w5809]
                  tunnel: w5795 -> [_ w5808]
                  tunnel: w5794 -> [_ w5807]
                  tunnel: w5793 -> [_ w5806]
                  tunnel: w5792 -> [_ w5805]
                  tunnel: w5791 -> [_ w5804]
                  tunnel: w5790 -> [_ w5803]
                  tunnel: w5789 -> [_ w5802]
                  frame False {
                  }
                  frame True {
                    n3196 = stacked-sequence {
                      tunnel: w5814 -> [_ w5827 w5872 w5917 w5962 w6007 _]
                      tunnel: w5813 -> [_ w5826 w5871 w5916 w5961 w6006 _]
                      tunnel: w5812 -> [_ w5816 _ _ _ _ _]
                      tunnel: w5811 -> [_ w5821 w5870 w5915 w5960 w6005 _]
                      tunnel: w5810 -> [_ w5815 _ _ _ _ _]
                      tunnel: w5809 -> [_ _ w5861 _ _ _ _]
                      tunnel: w5808 -> [_ _ w5860 _ _ _ _]
                      tunnel: w5807 -> [_ _ _ w5906 _ _ _]
                      tunnel: w5806 -> [_ _ _ w5905 _ _ _]
                      tunnel: w5805 -> [_ _ _ _ w5951 _ _]
                      tunnel: w5804 -> [_ _ _ _ w5950 _ _]
                      tunnel: w5803 -> [_ _ _ _ _ w5996 _]
                      tunnel: w5802 -> [_ _ _ _ _ w5995 _]
                      frame #0 {
                      }
                      frame #1 {
                        n3197 = case shown="False" w5827 {
                          tunnel: [w5858 w5859] -> w5843
                          tunnel: w5826 -> [_ w5859]
                          frame False {
                            n3198 = local read "CAL LAB01"() -> (w5858:T14)
                          }
                          frame True {
                          }
                        }
                        n3199 = local read "TEMP LA01"() -> (w5834:T9)
                        n3200 = local read "LAB01 TEMP"() -> (w5833:T12)
                        n3201 = call "sub vi - temperature delay v4.vi"("2-run"=w5815, "1-run"=w5816, "temp values IN"=w5834, "temp signals"=w5833) -> ("T2-N"=w5829:dbl, "T2-L"=w5830:dbl, "T1-N"=w5831:dbl, "T1-L"=w5832:dbl, "temp values OUT"=w5828:T44)  [unwired: 3 in]
                        n3202 = Unbundle By Name(w5843) -> ("1 (TL) cal"=w5838:dbl, "1 (TN) cal"=w5837:dbl, "2 (TL) cal"=w5836:dbl, "2 (TN) cal"=w5835:dbl)  [unwired: 6 out]
                        n3203 = local write "TEMP LA01"(w5828) -> ()
                        n3204 = Multiply(x=w5832, y=w5838) -> (x*y=w5825:dbl)
                        n3205 = Multiply(x=w5831, y=w5837) -> (x*y=w5823:dbl)
                        n3206 = Multiply(x=w5830, y=w5836) -> (x*y=w5820:dbl)
                        n3207 = Multiply(x=w5829, y=w5835) -> (x*y=w5819:dbl)
                        n3208 = case shown="True" w5816 {
                          tunnel: w5825 -> [w5852 w5857]
                          tunnel: w5821 -> [_ w5855]
                          tunnel: [w5852 w5856] -> w5824
                          tunnel: w5823 -> [w5851 w5854]
                          tunnel: [w5851 w5853] -> w5822
                          frame False {
                          }
                          frame True {
                            n3209 = Multiply(x=w5855, y=w5854) -> (x*y=w5853:dbl)
                            n3210 = Multiply(x=w5855, y=w5857) -> (x*y=w5856:dbl)
                          }
                        }
                        n3211 = case shown="True" w5815 {
                          tunnel: w5820 -> [w5845 w5850]
                          tunnel: w5821 -> [_ w5848]
                          tunnel: [w5845 w5849] -> w5818
                          tunnel: w5819 -> [w5844 w5847]
                          tunnel: [w5844 w5846] -> w5817
                          frame False {
                          }
                          frame True {
                            n3212 = Multiply(x=w5848, y=w5847) -> (x*y=w5846:dbl)
                            n3213 = Multiply(x=w5848, y=w5850) -> (x*y=w5849:dbl)
                          }
                        }
                        n3214 = local read "SIG LAB01-2"() -> (w5840:T2)
                        n3215 = local read "SIG LAB01-1"() -> (w5842:T2)
                        n3216 = Bundle By Name(cluster=w5842, "Tmp Live"=w5824, "Tmp Neut"=w5822) -> (w5841:T2)
                        n3217 = Bundle By Name(cluster=w5840, "Tmp Live"=w5818, "Tmp Neut"=w5817) -> (w5839:T2)
                        n3218 = local write "SIG LAB01-1"(w5841) -> ()
                        n3219 = local write "SIG LAB01-2"(w5839) -> ()
                      }
                      frame #2 {
                        n3220 = case shown="True" w5872 {
                          tunnel: [w5903 w5904] -> w5888
                          tunnel: w5871 -> [_ w5904]
                          frame False {
                            n3221 = local read "CAL LAB02"() -> (w5903:T15)
                          }
                          frame True {
                          }
                        }
                        n3222 = local read "LAB02 TEMP"() -> (w5879:T12)
                        n3223 = local read "TEMP LA02"() -> (w5878:T9)
                        n3224 = call "sub vi - temperature delay v4.vi"("2-run"=w5860, "1-run"=w5861, "temp values IN"=w5878, "temp signals"=w5879) -> ("T2-N"=w5873:dbl, "T2-L"=w5874:dbl, "T1-N"=w5875:dbl, "T1-L"=w5876:dbl, "temp values OUT"=w5877:T44)  [unwired: 3 in]
                        n3225 = Unbundle By Name(w5888) -> ("1 (TL) cal"=w5883:dbl, "1 (TN) cal"=w5882:dbl, "2 (TL) cal"=w5881:dbl, "2 (TN) cal"=w5880:dbl)  [unwired: 6 out]
                        n3226 = local write "TEMP LA02"(w5877) -> ()
                        n3227 = Multiply(x=w5876, y=w5883) -> (x*y=w5869:dbl)
                        n3228 = Multiply(x=w5875, y=w5882) -> (x*y=w5868:dbl)
                        n3229 = Multiply(x=w5874, y=w5881) -> (x*y=w5865:dbl)
                        n3230 = Multiply(x=w5873, y=w5880) -> (x*y=w5864:dbl)
                        n3231 = case shown="True" w5861 {
                          tunnel: w5869 -> [w5897 w5902]
                          tunnel: w5870 -> [_ w5900]
                          tunnel: [w5897 w5901] -> w5867
                          tunnel: w5868 -> [w5896 w5899]
                          tunnel: [w5896 w5898] -> w5866
                          frame False {
                          }
                          frame True {
                            n3232 = Multiply(x=w5900, y=w5899) -> (x*y=w5898:dbl)
                            n3233 = Multiply(x=w5900, y=w5902) -> (x*y=w5901:dbl)
                          }
                        }
                        n3234 = case shown="True" w5860 {
                          tunnel: w5865 -> [w5890 w5895]
                          tunnel: w5870 -> [_ w5893]
                          tunnel: [w5890 w5894] -> w5863
                          tunnel: w5864 -> [w5889 w5892]
                          tunnel: [w5889 w5891] -> w5862
                          frame False {
                          }
                          frame True {
